vi "Channel Basics Lesson 7.vi"() -> ()   [LabVIEW 2023]
doc: "This VI demonstrates that some channels can be forked and others cannot be forked."
uses:
  <vilib>/ChannelSupport/Channel Message/Channel Message.lvclass
  <extravilib>/ChannelInstances/Tag-i32/Read With Abort.vi
  <extravilib>/ChannelInstances/Stream-i32/Read With Abort.vi
  <extravilib>/ChannelInstances/Messenger-class'Channel Message'/Write With Abort.vi
  <extravilib>/ChannelInstances/Messenger-class'Channel Message'/Read With Abort.vi
  <extravilib>/ChannelInstances/Stream-i32/Write With Abort.vi
  <extravilib>/ChannelInstances/Tag-i32/Write With Abort.vi
  <extravilib>/ChannelInstances/Stream-i32/EndpointRead.vi
  <extravilib>/ChannelInstances/Stream-i32/Endpoint.vi
  <extravilib>/ChannelInstances/Messenger-class'Channel Message'/Instantiate.vi
  <extravilib>/ChannelInstances/Messenger-class'Channel Message'/Endpoint.vi
  <extravilib>/ChannelInstances/Stream-i32/Instantiate.vi
  <extravilib>/ChannelInstances/Stream-i32/)Channel.vi
  <resource>/ChannelSupport/_ChannelSupport/WaitIfNeeded.vi
  <extravilib>/ChannelInstances/Tag-i32/Instantiate.vi
  <extravilib>/ChannelInstances/Tag-i32/Endpoint.vi
  <extravilib>/ChannelInstances/Tag-i32/EndpointRead.vi
  <extravilib>/ChannelInstances/Tag-i32.lvlib
  <extravilib>/ChannelInstances/Stream-i32.lvlib
  <extravilib>/ChannelInstances/Messenger-class'Channel Message'.lvlib
panel:
  out "Messages Received":refnum<class "Channel Message.lvclass">[](array[class])
  out "element 5":i32
  out "element 4":i32
  out "element 7":i32
  out "element 6":i32
  out "element 3":i32
  out "element 2":i32
  out "element 1":i32
  # "Overview: This VI demonstrates that some channels can be forked and others cannot be forked.\n\nInstructions:\n1. Open the block diagram. Review the lessons presented there.\n2. Run the VI and observe the results of the different channel protocols."
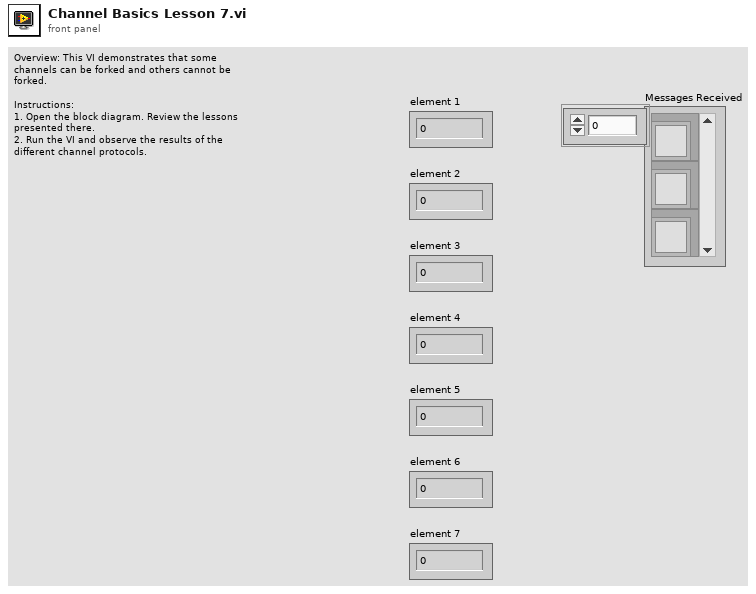
[diagram p1: front panel]
types:
  T1 = typedef "Stream-i32.lvlib/)Channel.ctl" = refnum<queue>
  T2 = typedef "Tag-i32.lvlib/))Channel.ctl" = refnum<queue>
  T3 = typedef "Messenger-class'Channel Message'.lvlib/))Channel.ctl" = refnum<queue>
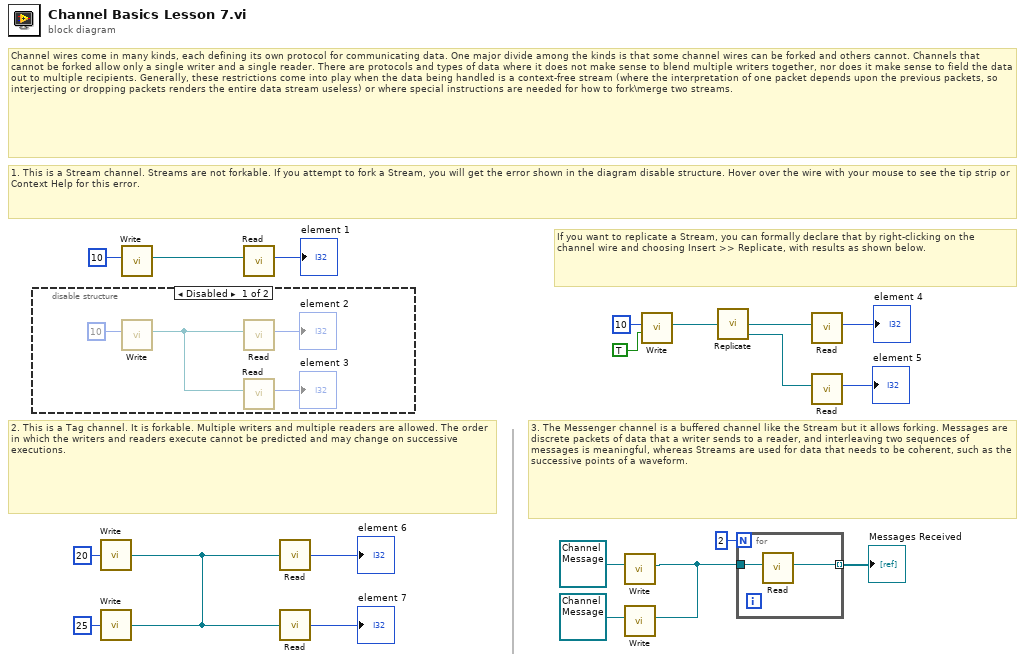
[diagram p0: block diagram]
diagram:
  # "If you want to replicate a Stream, you can formally declare that by right-clicking on the channel wire and choosing Insert >> Replicate, with results as shown below."
  # "3. The Messenger channel is a buffered channel like the Stream but it allows forking. Messages are discrete packets of data that a writer sends to a reader, and interleaving two sequences of messages is meaningful, whereas Streams are used for data that needs to be coherent, such as the successive points of a waveform."
  # "2. This is a Tag channel. It is forkable. Multiple writers and multiple readers are allowed. The order in which the writers and readers execute cannot be predicted and may change on successive executions."
  # "1. This is a Stream channel. Streams are not forkable. If you attempt to fork a Stream, you will get the error shown in the diagram disable structure. Hover over the wire with your mouse to see the tip strip or Context Help for this error."
  # "Channel wires come in many kinds, each defining its own protocol for communicating data. One major divide among the kinds is that some channel wires can be forked and others cannot. Channels that cannot be forked allow only a single writer and a single reader. There are protocols and types of data where it does not make sense to blend multiple writers together, nor does it make sense to field the data out to multiple recipients. Generally, these restrictions come into play when the data being handled is a context-free stream (where the interpretation of one packet depends upon the previous packets, so interjecting or dropping packets renders the entire data stream useless) or where special instructions are needed for how to fork\\merge two streams."
  n1 = disable-structure shown="Disabled" {
    frame Disabled {
      n2 = call <extravilib>:"Write.vi"("element"=10) -> ("channel"=w21:T1)  [unwired: 8 in, 2 out]
      n3 = call <extravilib>:"Read.vi"("channel"=w21) -> ("element"=→"element 2":i32)  [unwired: 6 in, 4 out]
      n4 = call <extravilib>:"Read.vi"("channel"=w21) -> ("element"=→"element 3":i32)  [unwired: 6 in, 4 out]
    }
    frame Enabled {
    }
  }
  n5 = call <extravilib>:"Write.vi"("element"=25) -> ("channel"=w20:T2)  [unwired: 1 out]
  n6 = call <extravilib>:"Write.vi"("element"=20, "channel"=w20) -> ()  [unwired: 1 out]
  n7 = call <extravilib>:"Write.vi"("element"=10) -> ("channel"=w14:T1)  [unwired: 8 in, 2 out]
  n8 = call <extravilib>:"Read.vi"("channel"=w14) -> ("element"=→"element 1":i32)  [unwired: 6 in, 4 out]
  n9 = call <extravilib>:"Read.vi"("channel"=w20) -> ("element"=→"element 6":i32)  [unwired: 1 in, 1 out]
  n10 = call <extravilib>:"Read.vi"("channel"=w20) -> ("element"=→"element 7":i32)  [unwired: 1 in, 1 out]
  n11 = call <extravilib>:"Write.vi"("element"=refnum<class "Channel Message.lvclass"> refnum ("Channel Message")) -> ("channel"=w1:T3)  [unwired: 8 in, 2 out]
  n12 = call <extravilib>:"Write.vi"("channel"=w1, "element"=refnum<class "Channel Message.lvclass"> refnum ("Channel Message")) -> ()  [unwired: 8 in, 2 out]
  n13 = call <extravilib>:"Write.vi"("last element? (F)"=TRUE, "element"=10) -> ("channel"=w11:T1)  [unwired: 7 in, 2 out]
  n14 = call <extravilib>:"Replicate.vi"("stream"=w11) -> ("stream copy 1"=w7:T1, "stream copy 2"=w8:T1)  [unwired: 7 in]
  n15 = for {
    N: 2 -> [_]
    tunnel: w1 -> [w26]
    tunnel: [w25] -> w4 mode=indexing
    n16 = call <extravilib>:"Read.vi"("channel"=w26) -> ("element"=w25:refnum<class "Channel Message.lvclass">)  [unwired: 8 in, 2 out]
  }
  "Messages Received" <- w4
  n17 = call <extravilib>:"Read.vi"("channel"=w7) -> ("element"=→"element 4":i32)  [unwired: 6 in, 4 out]
  n18 = call <extravilib>:"Read.vi"("channel"=w8) -> ("element"=→"element 5":i32)  [unwired: 6 in, 4 out]
